vi "Stepper.vi"() -> ()   [LabVIEW 2013]
uses:
  <vilib>/myRIO/Instrument Drivers/Onboard IO/DIO/vis/Smart Open.vi
  <vilib>/myRIO/Instrument Drivers/Onboard IO/DIO/vis/Write.vi
  <vilib>/myRIO/Common/Instrument Driver Framework/myRIO v1.0/UART/vis/myRIO v1.0 Close UART.vi
  <vilib>/myRIO/Instrument Drivers/Onboard IO/DIO/vis/Open.vi
  <vilib>/myRIO/Common/Instrument Driver Framework/myRIO v1.0/DIO/vis/myRIO v1.1 Open DIO.vi
  <vilib>/myRIO/Common/Instrument Driver Framework/Utilities/vis/Validate Channels.vi
  <vilib>/myRIO/Common/Instrument Driver Framework/myRIO v1.0/DIO/vis/myRIO v1.0 Reserve DIO.vi
  <vilib>/myRIO/Common/Instrument Driver Framework/myRIO v1.0/Resource Manager/vis/myRIO v1.0 Reserve Channel List.vi
  <vilib>/myRIO/Common/Instrument Driver Framework/myRIO v1.0/DIO/vis/myRIO v1.0 Build MUX Configuration DIO.vi
  <vilib>/myRIO/Common/Instrument Driver Framework/myRIO v1.0/Resource Manager/vis/myRIO v1.0 Reserve Channel.vi
  <vilib>/myRIO/Common/Instrument Driver Framework/myRIO v1.0/Resource Manager/vis/myRIO v1.0 Unreserve Channel.vi
  <vilib>/myRIO/Common/Instrument Driver Framework/myRIO v1.0/Resource Manager/vis/myRIO v1.0 Create Configuration List.vi
  <vilib>/myRIO/Common/Instrument Driver Framework/myRIO v1.0/Resource Manager/vis/myRIO v1.0 Build Mutex Name.vi
  <vilib>/myRIO/Common/Instrument Driver Framework/myRIO v1.0/myRIO v1.1 Open.vi
  <vilib>/Utility/VariantDataType/GetNumericInfo.vi
  <vilib>/Utility/error.llb/Error Cluster From Error Code.vi
  <vilib>/myRIO/Common/Instrument Driver Framework/Utilities/vis/IO Manager.vi
  <vilib>/myRIO/Common/Instrument Driver Framework/Utilities/vis/Configuration Manager.vi
  <vilib>/myRIO/Common/Instrument Driver Framework/myRIO v1.0/Resource Manager/vis/myRIO v1.0 Configure IO.vi
  <vilib>/myRIO/Common/Instrument Driver Framework/myRIO v1.0/myRIO v1.0 Close.vi
  <vilib>/myRIO/Common/Instrument Driver Framework/myRIO v1.0/DIO/vis/myRIO v1.0 Write DIO.vi
  <vilib>/myRIO/Common/Instrument Driver Framework/Utilities/vis/FPGA Ref Manager.vi
  <vilib>/myRIO/Common/Instrument Driver Framework/myRIO v1.0/myRIO v1.0 Reset FPGA.vi
  <vilib>/myRIO/Instrument Drivers/Utilities/Utilities.lvlib
panel:
  out "Z- 2":bool
  out "Z+ 2":bool
  out "Y- 2":bool
  out "Y+ 2":bool
  out "X- 2":bool
  out "X+ 2":bool
  out "Z:":dbl
  out "Y:":dbl
  out "X:":dbl
  in  "z, step/mm":dbl=320.0
  in  "y, step/mm":dbl=40.02
  in  "x, step/mm":dbl=40.02
  in  "Step Size (mm)":u32=1
  out "Dir Z":bool
  out "Dir Y":bool
  out "Pulse Z":bool
  out "Pulse Y":bool
  in  "Z-":bool
  in  "Z+":bool
  in  "Time (ms)":u32=1
  out "Dir X":bool
  out "Enable":bool
  in  "Y-":bool
  in  "Y+":bool
  in  "X+":bool
  in  "X-":bool
  out "Pulse X":bool
  out "error out":errorcluster
  in  "Stop Button":bool
  # "Manual Location:"
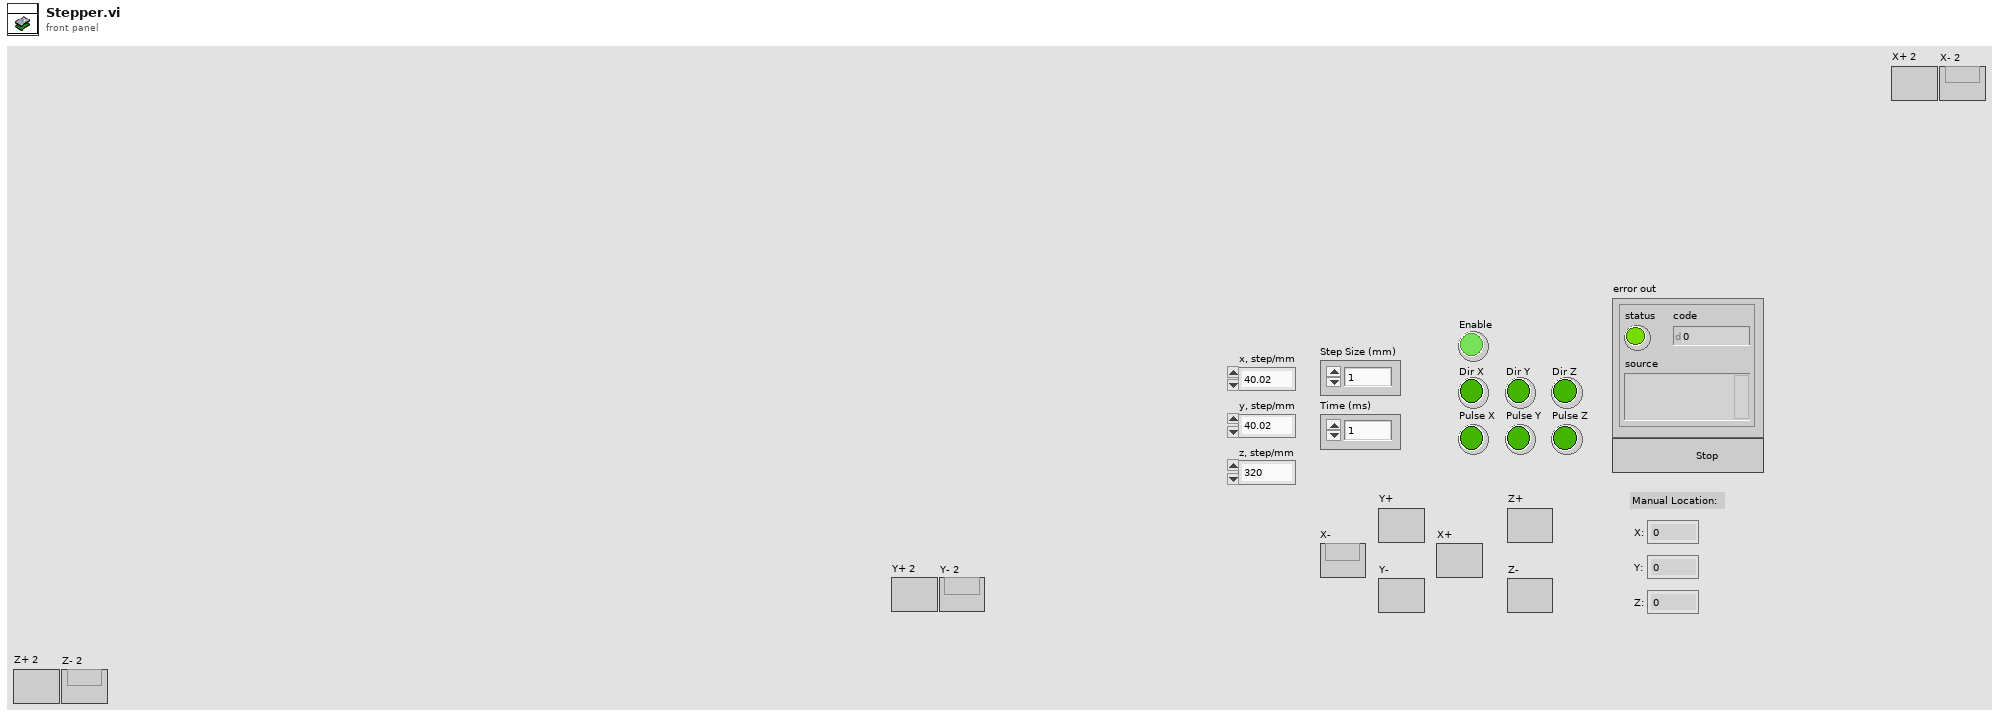
[diagram p1: front panel]
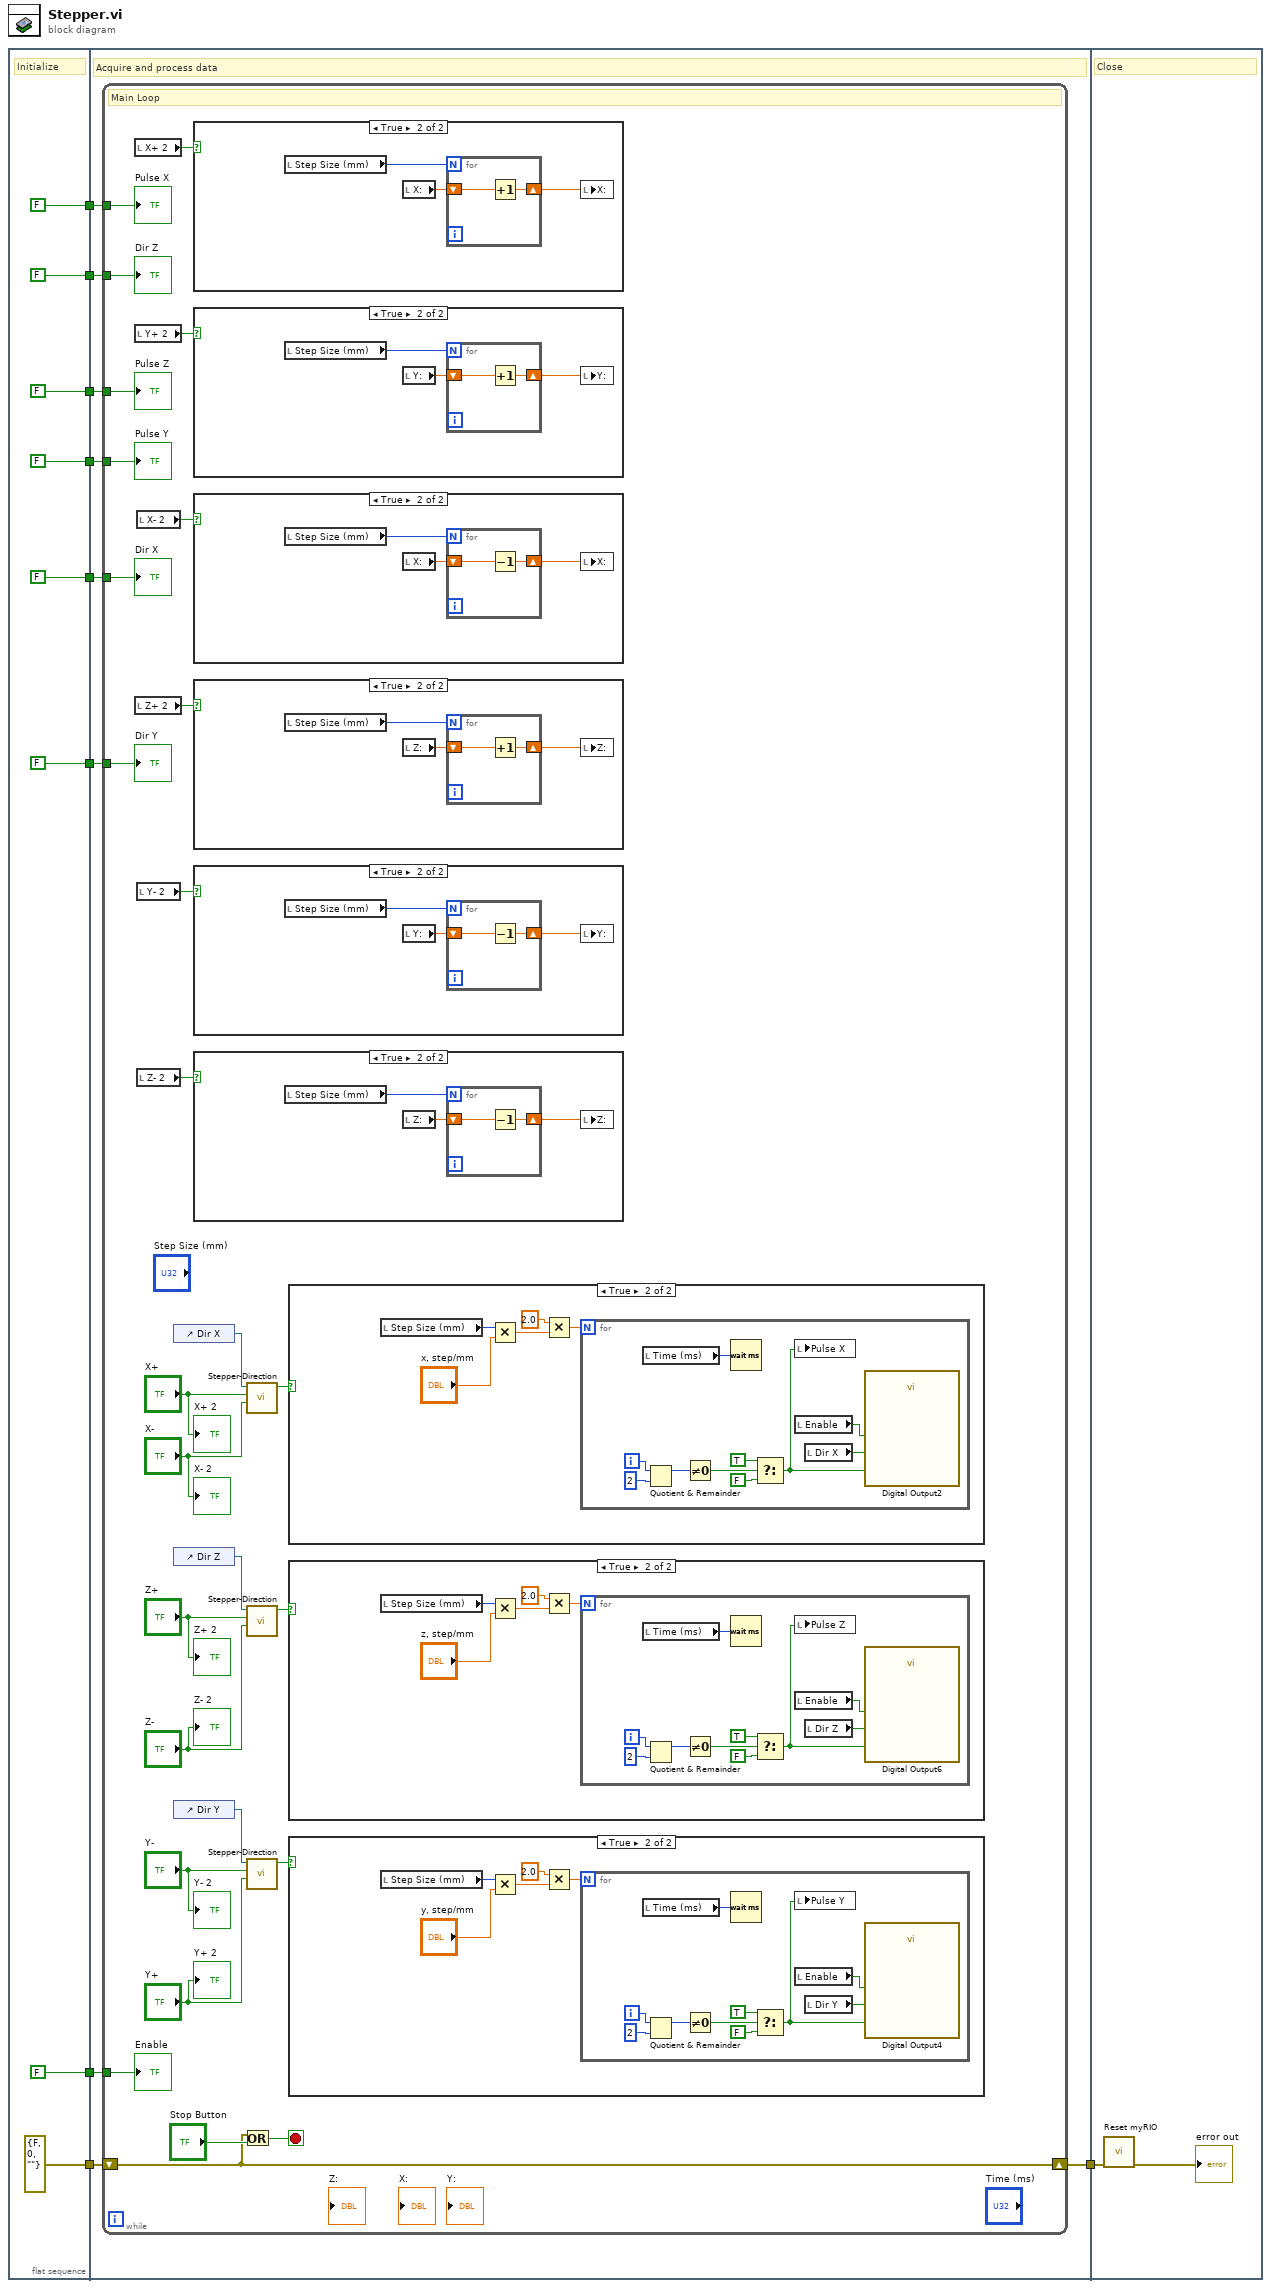
[diagram p0: block diagram]
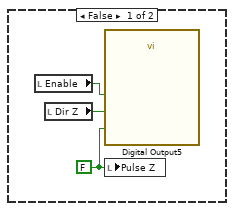
[diagram p8: hidden frame]
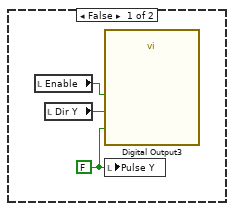
[diagram p9: hidden frame]
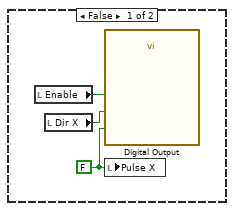
[diagram p10: hidden frame]
diagram:
  n1 = flat-sequence {
    tunnel: [errorcluster {"status"=FALSE, "code"=0, "source"=""} ("error out")] -> w9
    tunnel: [FALSE] -> w7
    tunnel: [FALSE] -> w6
    tunnel: [FALSE ("Pulse X")] -> w5
    tunnel: [FALSE ("Pulse X")] -> w4
    tunnel: [FALSE] -> w3
    tunnel: [FALSE ("Pulse X")] -> w2
    tunnel: [FALSE] -> w1
    tunnel: w9 -> [w26]
    tunnel: [w25] -> w8
    tunnel: w7 -> [w24]
    tunnel: w6 -> [w23]
    tunnel: w5 -> [w22]
    tunnel: w4 -> [w21]
    tunnel: w3 -> [w20]
    tunnel: w2 -> [w19]
    tunnel: w1 -> [w18]
    tunnel: w8 -> [w140]
    frame #0 {
      # "Initialize"
    }
    frame #1 {
      # "Acquire and process data"
      n2 = while {
        shift-right: [w52] -> w25
        shift-left: w26 -> [w52]
        tunnel: w24 -> [w51]
        tunnel: w23 -> [w50]
        tunnel: w22 -> [w49]
        tunnel: w21 -> [w48]
        tunnel: w20 -> [w47]
        tunnel: w19 -> [w46]
        tunnel: w18 -> [w45]
        stop <- w53 stop-if-true
        # "Main Loop"
        n3 = local read "X+ 2"() -> (w37:bool)
        n4 = local read "Y+ 2"() -> (w28:bool)
        n5 = local read "Z+ 2"() -> (w30:bool)
        n6 = local read "X- 2"() -> (w38:bool)
        n7 = local read "Y- 2"() -> (w27:bool)
        n8 = local read "Z- 2"() -> (w29:bool)
        n9 = control-ref of="Dir X"() -> (w42:refnum<vi>)
        n10 = control-ref of="Dir Z"() -> (w39:refnum<vi>)
        n11 = control-ref of="Dir Y"() -> (w43:refnum<vi>)
        n12 = case shown="True" w37 {
          frame False {
          }
          frame True {
            n13 = local read "Step Size (mm)"() -> (w81:u32)
            n14 = local read "X:"() -> (w80:dbl)
            n15 = for {
              N: w81 -> [_]
              shift-right: [w83] -> w82
              shift-left: w80 -> [w84]
              n16 = Increment(x=w84) -> (x+1=w83:dbl)
            }
            n17 = local write "X:"(w82) -> ()
          }
        }
        n18 = case shown="True" w28 {
          frame False {
          }
          frame True {
            n19 = local read "Step Size (mm)"() -> (w61:u32)
            n20 = local read "Y:"() -> (w60:dbl)
            n21 = for {
              N: w61 -> [_]
              shift-right: [w63] -> w62
              shift-left: w60 -> [w64]
              n22 = Increment(x=w64) -> (x+1=w63:dbl)
            }
            n23 = local write "Y:"(w62) -> ()
          }
        }
        n24 = case shown="True" w38 {
          frame False {
          }
          frame True {
            n25 = local read "Step Size (mm)"() -> (w76:u32)
            n26 = local read "X:"() -> (w77:dbl)
            n27 = for {
              N: w76 -> [_]
              shift-right: [w78] -> w75
              shift-left: w77 -> [w79]
              n28 = Decrement(x=w79) -> (x-1=w78:dbl)
            }
            n29 = local write "X:"(w75) -> ()
          }
        }
        n30 = case shown="True" w30 {
          frame False {
          }
          frame True {
            n31 = local read "Step Size (mm)"() -> (w71:u32)
            n32 = local read "Z:"() -> (w70:dbl)
            n33 = for {
              N: w71 -> [_]
              shift-right: [w73] -> w72
              shift-left: w70 -> [w74]
              n34 = Increment(x=w74) -> (x+1=w73:dbl)
            }
            n35 = local write "Z:"(w72) -> ()
          }
        }
        n36 = case shown="True" w27 {
          frame False {
          }
          frame True {
            n37 = local read "Step Size (mm)"() -> (w56:u32)
            n38 = local read "Y:"() -> (w57:dbl)
            n39 = for {
              N: w56 -> [_]
              shift-right: [w58] -> w55
              shift-left: w57 -> [w59]
              n40 = Decrement(x=w59) -> (x-1=w58:dbl)
            }
            n41 = local write "Y:"(w55) -> ()
          }
        }
        n42 = case shown="True" w29 {
          frame False {
          }
          frame True {
            n43 = local read "Step Size (mm)"() -> (w66:u32)
            n44 = local read "Z:"() -> (w67:dbl)
            n45 = for {
              N: w66 -> [_]
              shift-right: [w68] -> w65
              shift-left: w67 -> [w69]
              n46 = Decrement(x=w69) -> (x-1=w68:dbl)
            }
            n47 = local write "Z:"(w65) -> ()
          }
        }
        n48 = Or(x=w52, y="Stop Button") -> (x .or. y?=w53:bool)
        n49 = call "Stepper-Direction.vi"("+Axis"="X-", "-Axis"="X+", "Boolean in"=w42) -> ("Boolean"=w41:bool)  [unwired: 8 in]
        n50 = call "Stepper-Direction.vi"("+Axis"="Z-", "-Axis"="Z+", "Boolean in"=w39) -> ("Boolean"=w40:bool)  [unwired: 8 in]
        n51 = call "Stepper-Direction.vi"("+Axis"="Y+", "-Axis"="Y-", "Boolean in"=w43) -> ("Boolean"=w44:bool)  [unwired: 8 in]
        n52 = case shown="True" w41 {
          frame False {
            w121 = FALSE
            n53 = local read "Enable"() -> (w123:bool)
            n54 = local read "Dir X"() -> (w122:bool)
            n55 = call "Digital Output"("Enable (A/DIO8 (Pin 27))"=w123, "Dir X (A/DIO5 (Pin 21))"=w122, "Pulse X (A/DIO2 (Pin 15))"=w121) -> ()  [unwired: 24 in, 1 out]
            n56 = local write "Pulse X"(w121) -> ()
          }
          frame True {
            n57 = local read "Step Size (mm)"() -> (w128:u32)
            n58 = Multiply(x=w128, y="x, step/mm") -> (x*y=w125:dbl)
            n59 = Multiply(x=2.0, y=w125) -> (x*y=w126:dbl)
            n60 = for {
              N: w126 -> [_]
              i -> [w138]
              n61 = local read "Time (ms)"() -> (w129:u32)
              n62 = Quotient & Remainder(x=w138, y=2) -> (x-y*floor(x/y)=w136:i32)  [unwired: 1 out]
              n63 = Not Equal To 0?(x=w136) -> (x != 0?=w135:bool)
              n64 = Wait (ms)(milliseconds to wait=w129) -> ()  [unwired: 1 out]
              n65 = Select(t=TRUE, s=w135, f=FALSE) -> (s? t:f=w130:bool)
              n66 = local write "Pulse X"(w130) -> ()
              n67 = local read "Enable"() -> (w132:bool)
              n68 = local read "Dir X"() -> (w131:bool)
              n69 = call "Digital Output2"("Enable (A/DIO8 (Pin 27))"=w132, "Dir X (A/DIO5 (Pin 21))"=w131, "Pulse X (A/DIO2 (Pin 15))"=w130) -> ()  [unwired: 24 in, 1 out]
            }
          }
        }
        n70 = case shown="True" w40 {
          frame False {
            w85 = FALSE
            n71 = local read "Enable"() -> (w87:bool)
            n72 = local read "Dir Z"() -> (w86:bool)
            n73 = call "Digital Output5"("Enable (A/DIO8 (Pin 27))"=w87, "Dir Z (A/DIO7 (Pin 25))"=w86, "Pulse Z (A/DIO4 (Pin 19))"=w85) -> ()  [unwired: 24 in, 1 out]
            n74 = local write "Pulse Z"(w85) -> ()
          }
          frame True {
            n75 = local read "Step Size (mm)"() -> (w89:u32)
            n76 = Multiply(x=w89, y="z, step/mm") -> (x*y=w90:dbl)
            n77 = Multiply(x=2.0, y=w90) -> (x*y=w92:dbl)
            n78 = for {
              N: w92 -> [_]
              i -> [w102]
              n79 = local read "Time (ms)"() -> (w93:u32)
              n80 = Quotient & Remainder(x=w102, y=2) -> (x-y*floor(x/y)=w100:i32)  [unwired: 1 out]
              n81 = Not Equal To 0?(x=w100) -> (x != 0?=w99:bool)
              n82 = Wait (ms)(milliseconds to wait=w93) -> ()  [unwired: 1 out]
              n83 = Select(t=TRUE, s=w99, f=FALSE) -> (s? t:f=w94:bool)
              n84 = local write "Pulse Z"(w94) -> ()
              n85 = local read "Enable"() -> (w96:bool)
              n86 = local read "Dir Z"() -> (w95:bool)
              n87 = call "Digital Output6"("Enable (A/DIO8 (Pin 27))"=w96, "Dir Z (A/DIO7 (Pin 25))"=w95, "Pulse Z (A/DIO4 (Pin 19))"=w94) -> ()  [unwired: 24 in, 1 out]
            }
          }
        }
        n88 = case shown="True" w44 {
          frame False {
            w103 = FALSE
            n89 = local read "Enable"() -> (w105:bool)
            n90 = local read "Dir Y"() -> (w104:bool)
            n91 = call "Digital Output3"("Enable (A/DIO8 (Pin 27))"=w105, "Dir Y (A/DIO6 (Pin 23))"=w104, "Pulse Y (A/DIO3 (Pin 17))"=w103) -> ()  [unwired: 24 in, 1 out]
            n92 = local write "Pulse Y"(w103) -> ()
          }
          frame True {
            n93 = local read "Step Size (mm)"() -> (w107:u32)
            n94 = Multiply(x=w107, y="y, step/mm") -> (x*y=w108:dbl)
            n95 = Multiply(x=2.0, y=w108) -> (x*y=w110:dbl)
            n96 = for {
              N: w110 -> [_]
              i -> [w120]
              n97 = local read "Time (ms)"() -> (w111:u32)
              n98 = Quotient & Remainder(x=w120, y=2) -> (x-y*floor(x/y)=w118:i32)  [unwired: 1 out]
              n99 = Not Equal To 0?(x=w118) -> (x != 0?=w117:bool)
              n100 = Wait (ms)(milliseconds to wait=w111) -> ()  [unwired: 1 out]
              n101 = Select(t=TRUE, s=w117, f=FALSE) -> (s? t:f=w112:bool)
              n102 = local write "Pulse Y"(w112) -> ()
              n103 = local read "Enable"() -> (w114:bool)
              n104 = local read "Dir Y"() -> (w113:bool)
              n105 = call "Digital Output4"("Enable (A/DIO8 (Pin 27))"=w114, "Dir Y (A/DIO6 (Pin 23))"=w113, "Pulse Y (A/DIO3 (Pin 17))"=w112) -> ()  [unwired: 24 in, 1 out]
            }
          }
        }
        "Pulse X" <- w49
        "Enable" <- w51
        "Dir X" <- w50
        "Pulse Y" <- w47
        "Pulse Z" <- w48
        "Dir Y" <- w45
        "Dir Z" <- w46
        "X+ 2" <- "X+"
        "X- 2" <- "X-"
        "Y+ 2" <- "Y+"
        "Y- 2" <- "Y-"
        "Z+ 2" <- "Z+"
        "Z- 2" <- "Z-"
      }
    }
    frame #2 {
      # "Close"
      n106 = call <vilib>:"Reset myRIO.vi"("error in (no error)"=w140) -> ("error out"=→"error out":errorcluster)  [unwired: 10 in]
    }
  }
